vi "Command Wait.vi"(2 "Input Robot System Funtions":T1, 3 "Cmd Parameter 1":dbl, 4 "Cmd Parameter 2":dbl, 5 "Startup":bool) -> (0 "Robot System Functions":T1, 1 "Completed":bool)   [LabVIEW 2014]
uses:
  Subsystems VIs/Robot Commands.ctl
  Command Execution State.ctl
panel:
  # "Sample robot\ncontrol output.\nReplace with \nactual teleop \ncontrol signal \nstructure."
  # "Field Centric"
  # "Field Centric"
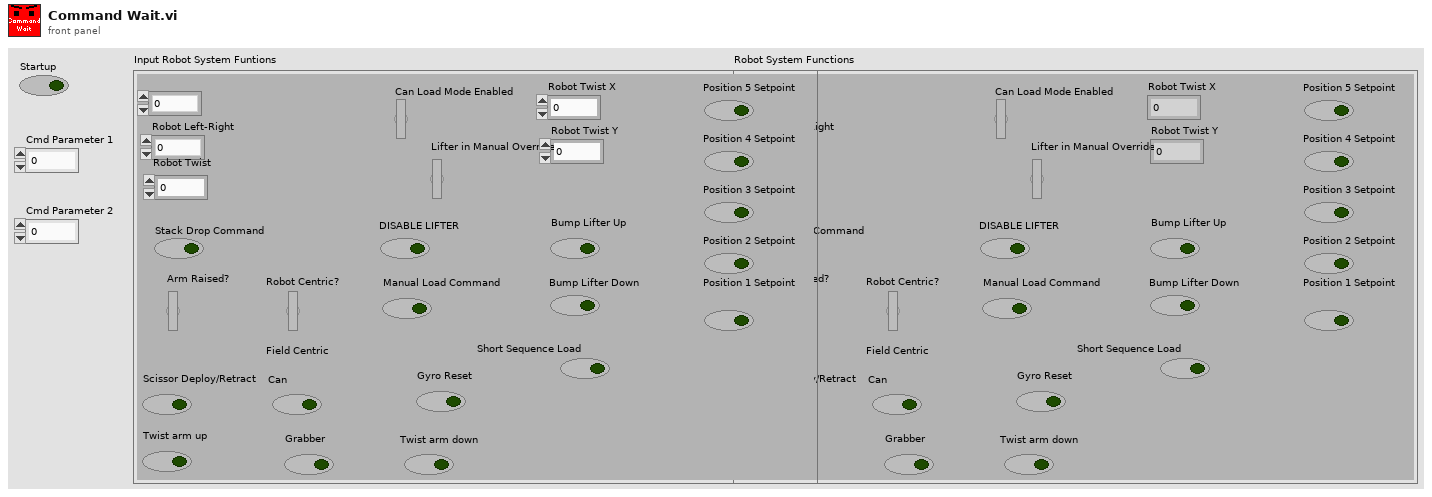
[diagram p1: front panel]
types:
  T1 = typedef "Robot Commands.ctl" = cluster{"Robot Forward-Reverse":dbl, "Robot Left-Right":dbl, "Robot Twist":dbl, "Can Load Mode Enabled":bool, "Lifter in Manual Override?":bool, "Stack Drop Command":bool, "Arm Raised?":bool, "DISABLE LIFTER":bool, "Position 1 Setpoint":bool, "Position 2 Setpoint":bool, "Position 3 Setpoint":bool, "Position 4 Setpoint":bool, "Position 5 Setpoint":bool, "Bump Lifter Down":bool, "Bump Lifter Up":bool, "Manual Load Command":bool, "Robot Centric?":bool, "Scissor Deploy/Retract":bool, "Grabber":bool, "Can":bool, "Twist arm up":bool, "Gyro Reset":bool, "Twist arm down":bool, "Short Sequence Load":bool, "Robot Twist X":dbl, "Robot Twist Y":dbl}
  T2 = typedef "Command Execution State.ctl" = enum16{"Initialize", "Execute", "Finish"}
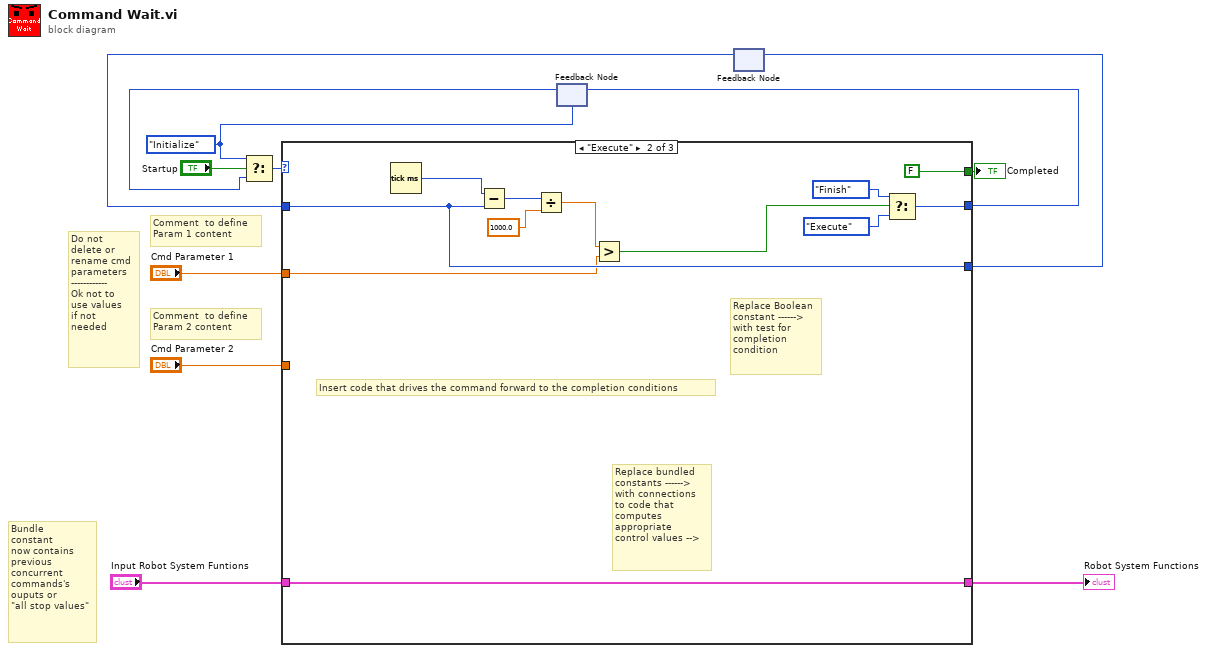
[diagram p0: block diagram]
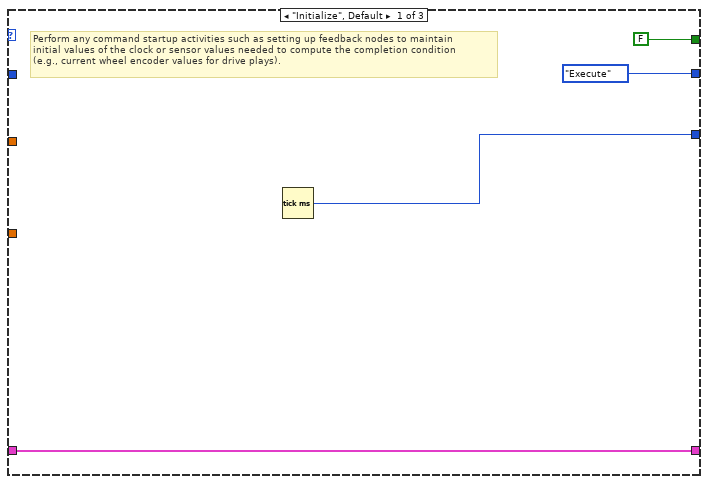
[diagram p2: hidden frame]
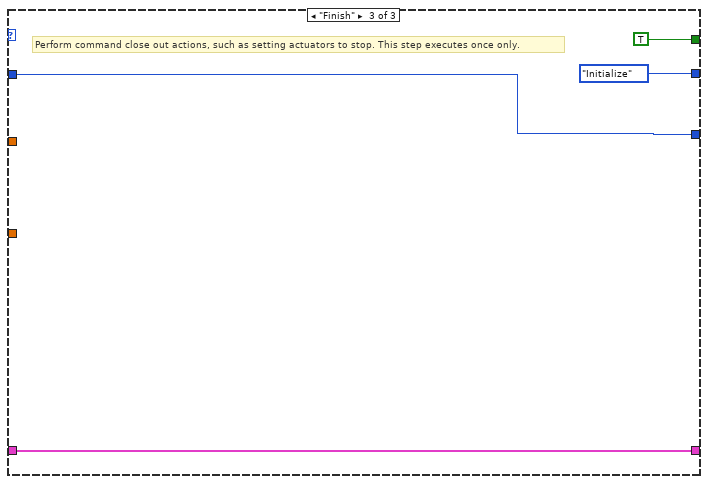
[diagram p3: hidden frame]
diagram:
  w7 = Command_Execution_State."Initialize" ("Play State")
  # "Bundle \nconstant\nnow contains\nprevious \nconcurrent\ncommands's\nouputs or\n\"all stop values\""
  # "Do not \ndelete or\nrename cmd\nparameters\n------------\nOk not to \nuse values\nif not \nneeded"
  # "Comment  to define\nParam 2 content"
  # "Comment  to define\nParam 1 content"
  n1 = feedback #1(w7) -> (w8:T2)
  n2 = Select(t=w7, s="Startup", f=w8) -> (s? t:f=w12:T2)
  n3 = feedback #2() -> (w3:u32)  [unwired: 1 in]
  n4 = case shown="\"Execute\"" w12 {
    tunnel: [FALSE FALSE TRUE] -> w10
    tunnel: [Command_Execution_State."Execute" ("Play State") w26 Command_Execution_State."Initialize" ("f")] -> w9
    tunnel: "Cmd Parameter 1" -> [_ w18 _]
    tunnel: "Cmd Parameter 2" -> [_ _ _]
    tunnel: [w14 w24 w30] -> w1
    tunnel: "Input Robot System Funtions" -> [w14 w24 w30]
    tunnel: [w13 w20 w29] -> w4
    tunnel: w3 -> [_ w20 w29]
    frame "Initialize", Default {
      # "Perform any command startup activities such as setting up feedback nodes to maintain \ninitial values of the clock or sensor values needed to compute the completion condition\n(e.g., current wheel encoder values for drive plays)."
      n5 = Tick Count (ms)() -> (millisecond timer value=w13:u32)
    }
    frame "Execute" {
      # "Replace bundled \nconstants ------>\nwith connections \nto code that\ncomputes \nappropriate \ncontrol values -->"
      # "Replace Boolean\nconstant ------>\nwith test for \ncompletion \ncondition"
      # "Insert code that drives the command forward to the completion conditions"
      n6 = Tick Count (ms)() -> (millisecond timer value=w23:u32)
      n7 = Subtract(x=w23, y=w20) -> (x-y=w21:u32)
      n8 = Divide(x=w21, y=1000.0) -> (x/y=w19:dbl)
      n9 = Greater?(x=w19, y=w18) -> (0:w17:bool)
      n10 = Select(t=Command_Execution_State."Finish" ("Play State"), s=w17, f=Command_Execution_State."Execute") -> (s? t:f=w26:T2)
    }
    frame "Finish" {
      # "Perform command close out actions, such as setting actuators to stop. This step executes once only."
    }
  }
  "Completed" <- w10
  "Robot System Functions" <- w1
  n11 = feedback-in #1(w9) -> ()
  n12 = feedback-in #2(w4) -> ()
